vi "get brake settings.vi"(8 "error in (no error)":errorcluster, 10 "brake_settings":T1, 11 "id":i32) -> (0 "error out":errorcluster, 2 "brake_settings out":T1, 3 "function return":i32)   [LabVIEW 2012, in "libximc.lvlib"]
doc: "result_t XIMC_API get_brake_settings (device_t id, brake_settings_t* brake_settings);"
uses:
  libximc.lvlib
  libximc.dll
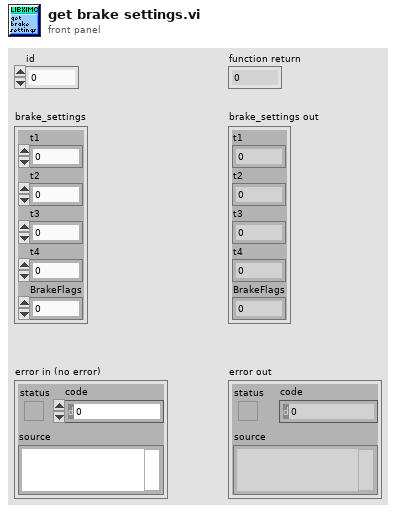
[diagram p1: front panel]
types:
  T1 = cluster{"t1":u32, "t2":u32, "t3":u32, "t4":u32, "BrakeFlags":u32}
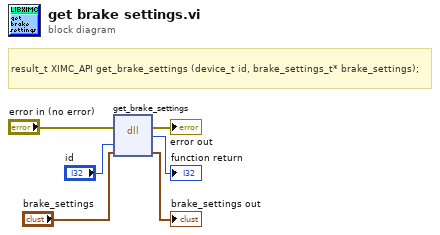
[diagram p0: block diagram]
diagram:
  # "result_t XIMC_API get_brake_settings (device_t id, brake_settings_t* brake_settings);"
  n1 = dll-call lib="C:/Users/user/Desktop/labview-2.9.11-gen/libximc.*" fn="get_brake_settings"(error in="error in (no error)", "id"="id", "brake_settings"="brake_settings") -> (error out=→"error out":errorcluster, →"function return":i32, "brake_settings"=→"brake_settings out":T1)  [unwired: 3 in, 1 out]
